vi "Play Path.vi"() -> ()   [LabVIEW 2020]
uses:
  Implementation/Drive Operations.ctl
  Implementation/Drive Setpoints.ctl
  Support Code/submodules/bordeaux-pathinator/Bordeaux/Types/Path Type.ctl
  Support Code/submodules/bordeaux-pathinator/Bordeaux/Types/Drive Type.ctl
  Support Code/submodules/bordeaux-pathinator/Bordeaux/Types/Angluar Limits.ctl
  Support Code/submodules/bordeaux-pathinator/Bordeaux/Types/Overrides.ctl
  <vilib>/picture/picture.llb/imagedata.ctl
  Support Code/submodules/bordeaux-pathinator/Bordeaux/Types/Single Cmd Info.ctl
panel:
  in  "Path Info":T7 {"Fields"."Overrides"."Angle Override" step=5.0; "Fields"."Overrides"."Velocity Override" step=5.0; "Fields"."Overrides"."Angular Override" step=5.0; "Fields"."Angular Limits"."Jerk (deg/s^3)" min=0.0 step=1.0; "Fields"."Angular Limits"."Accel (deg/s^2)" min=0.0; "Fields"."Angular Limits"."Velocity (deg/s)" min=0.0}
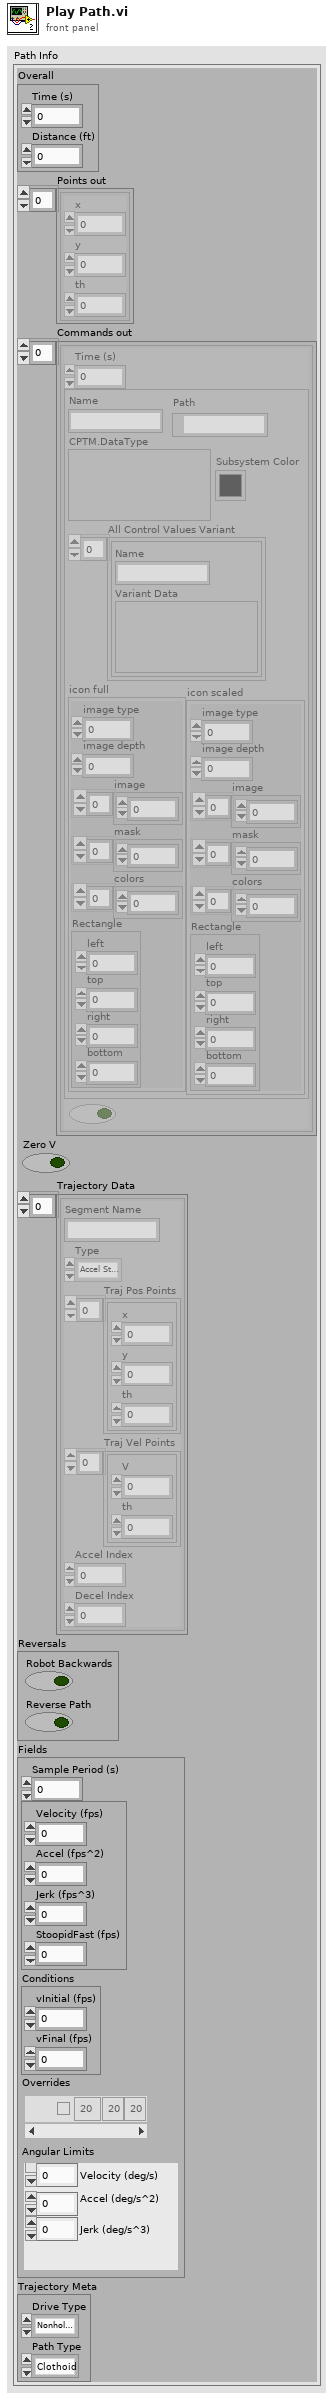
[diagram p1: front panel]
types:
  T1 = typedef "Single Cmd Info.ctl" = cluster{"Name":string, "CPTM.DataType":variant, "All Control Values Variant":cluster{"Name":string, "Variant Data":variant}[], "icon full":T2, "icon scaled":T2, "Path":path, "Subsystem Color":u32}
  T2 = typedef "imagedata.ctl" = cluster{"image type":i32, "image depth":i32, "image":u8[], "mask":u8[], "colors":u32[], "Rectangle":cluster{"left":i16, "top":i16, "right":i16, "bottom":i16}}
  T3 = typedef "Overrides.ctl" = cluster{"Count":string, "Angular Override":dbl, "Enabled?":bool, "Velocity Override":dbl, "Angle Override":dbl}[]
  T4 = typedef "Angluar Limits.ctl" = cluster{"Velocity (deg/s)":dbl, "Accel (deg/s^2)":dbl, "Jerk (deg/s^3)":dbl}
  T5 = typedef "Drive Type.ctl" = enum16{"Nonholonomic", "Holonomic"}
  T6 = typedef "Path Type.ctl" = enum16{"Clothoid", "Bezier"}
  T7 = cluster{"Overall":cluster{"Time (s)":dbl, "Distance (ft)":dbl}, "Points out":cluster{"x":dbl, "y":dbl, "th":dbl}[], "Commands out":cluster{"Time (s)":dbl, T1, bool}[], "Zero V":bool, "Trajectory Data":cluster{"Segment Name":string, "Type":enum16{"Accel Straight", "Const Straight", "Blend", "Circle"}, "Traj Pos Points":cluster{"x":dbl, "y":dbl, "th":dbl}[], "Traj Vel Points":cluster{"V":dbl, "th":dbl}[], "Accel Index":i32, "Decel Index":i32}[], "Reversals":cluster{"Robot Backwards":bool, "Reverse Path":bool}, "Fields":cluster{"Sample Period (s)":dbl, cluster{"Velocity (fps)":dbl, "Accel (fps^2)":dbl, "Jerk (fps^3)":dbl, "StoopidFast (fps)":dbl}, "Conditions":cluster{"vInitial (fps)":dbl, "vFinal (fps)":dbl}, "Overrides":T3, "Angular Limits":T4}, "Trajectory Meta":cluster{"Drive Type":T5, "Path Type":T6}}
  T8 = typedef "Drive Operations.ctl" = enum16{"Reserve", "Read Current", "Immediate", "Calibrate", "Play Path"}
  T9 = typedef "Drive Setpoints.ctl" = cluster{"Operation":T8, "Trans Vel":cluster{"x":dbl, "y":dbl}, "Rot Vel":cluster{"omega":dbl}, "Path Info":cluster{"Overall":cluster{"Time (s)":dbl, "Distance (ft)":dbl}, "Points out":cluster{"x":dbl, "y":dbl, "th":dbl}[], "Commands out":cluster{"Time (s)":dbl, T1, bool}[], "Zero V":bool, "Trajectory Data":cluster{"Segment Name":string, "Type":enum16{"Accel Straight", "Const Straight", "Blend", "Circle"}, "Traj Pos Points":cluster{"x":dbl, "y":dbl, "th":dbl}[], "Traj Vel Points":cluster{"V":dbl, "th":dbl}[], "Accel Index":i32, "Decel Index":i32}[], "Reversals":cluster{"Robot Backwards":bool, "Reverse Path":bool}, "Fields":cluster{"Sample Period (s)":dbl, cluster{"Velocity (fps)":dbl, "Accel (fps^2)":dbl, "Jerk (fps^3)":dbl, "StoopidFast (fps)":dbl}, "Conditions":cluster{"vInitial (fps)":dbl, "vFinal (fps)":dbl}, "Overrides":T3, "Angular Limits":T4}, "Trajectory Meta":cluster{"Drive Type":T5, "Path Type":T6}}}
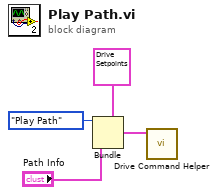
[diagram p0: block diagram]
diagram:
  n1 = Bundle(cluster=T9 {"Operation"=enum."Reserve", "Trans Vel"={"x"=0.0, "y"=0.0}, "Rot Vel"={"omega"=0.0}, "Path Info"={"Overall"={"Time (s)"=0.0, "Distance (ft)"=0.0}, "Points out"=[], "Commands out"=[], "Zero V"=FALSE, "Trajectory Data"=[], "Reversals"={"Robot Backwards"=FALSE, "Reverse Path"=FALSE}, "Fields"={"Sample Period (s)"=0.0, {"Velocity (fps)"=0.0, "Accel (fps^2)"=0.0, "Jerk (fps^3)"=0.0, "StoopidFast (fps)"=0.0}, "Conditions"={"vInitial (fps)"=0.0, "vFinal (fps)"=0.0}, "Overrides"=[], "Angular Limits"={"Velocity (deg/s)"=0.0, "Accel (deg/s^2)"=0.0, "Jerk (deg/s^3)"=0.0}}, "Trajectory Meta"={"Drive Type"=enum."Nonholonomic", "Path Type"=enum."Clothoid"}}} ("SubSystem Data"), "Operation"=Drive_Operations."Play Path", "Path Info"="Path Info") -> (w3:T9)  [unwired: 2 in]
  n2 = call "Drive Command Helper.vi"("SubSystem Data"=w3) -> ()  [unwired: 8 in, 3 out]
